vi "stimulate_and_record.vi"(3 "SSH password":string, 4 "Transfer and Run Date Folder After Experiment":bool, 5 "SSH user name":string, 6 "Tags":string, 7 "Frames":i32, 8 "Convert Power to Voltage":bool, 9 "voltages/power":dbl[](array[numeric]), 10 "parameters":string[](array[string]), 11 "parameters headers":string[](array[string])) -> ()   [LabVIEW 2014]
uses:
  <vilib>/userdefined/High Color/IMAQdx.ctl
  <vilib>/Utility/file.llb/Write To Spreadsheet File (string).vi
  <vilib>/Utility/file.llb/Read From Spreadsheet File (string).vi
  <vilib>/Utility/file.llb/Write To Spreadsheet File (DBL).vi
panel:
  out "Error":string
  out "Save Directory":path
  out "Buffer Number Out":u32
  out "Image":T1(plugin-control)
  in  "stop":bool
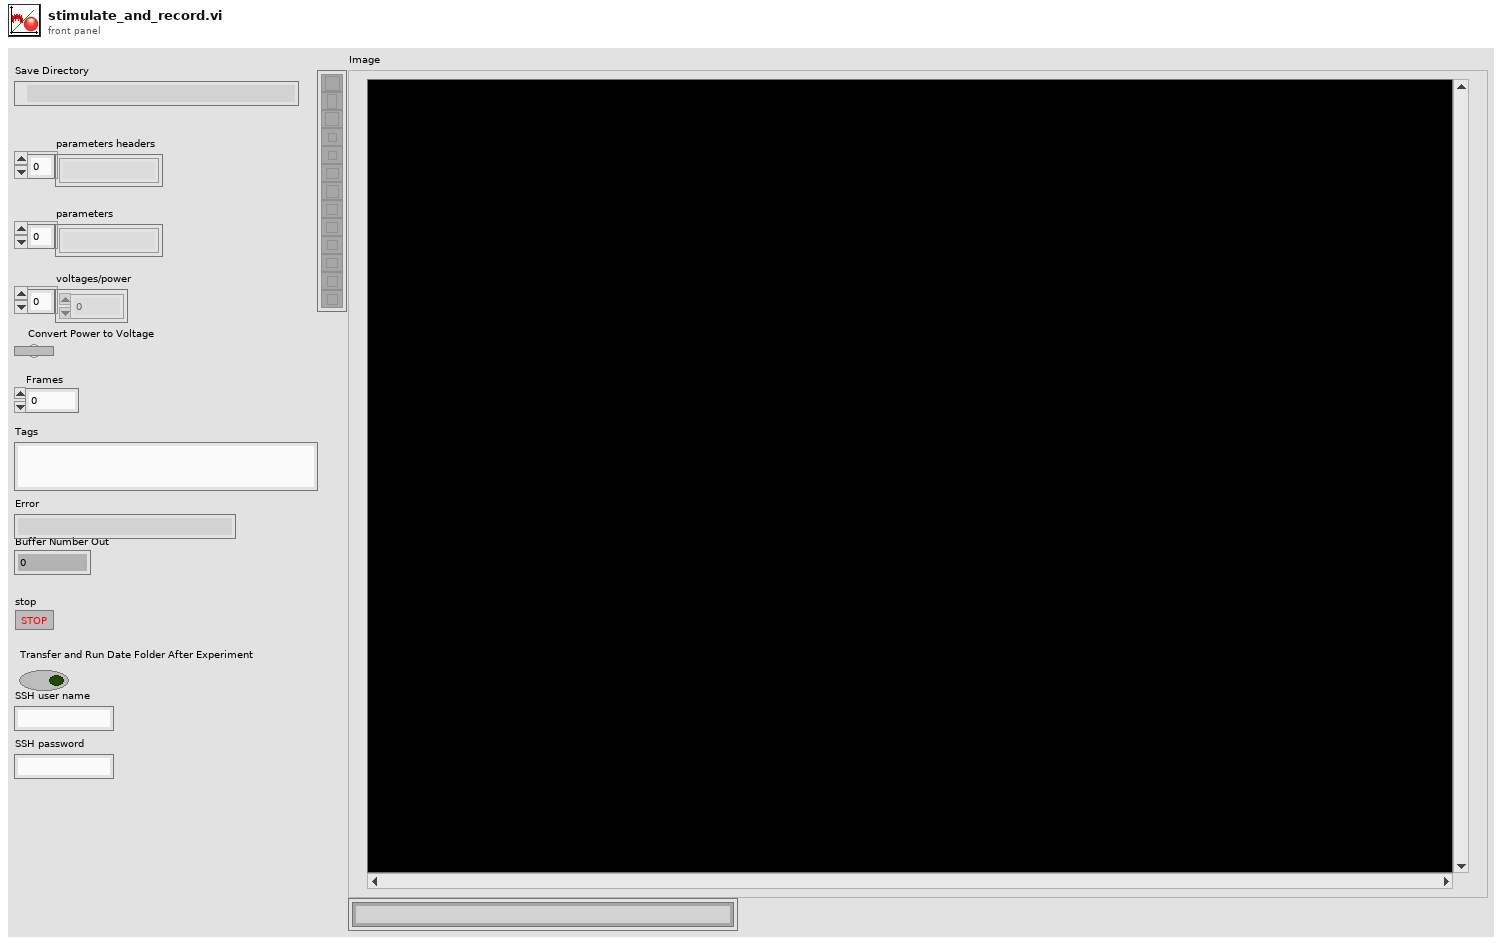
[diagram p1: front panel]
types:
  T1 = typedef "IMAQ Image.ctl" = refnum<image>
  T2 = typedef "IMAQdx.ctl" = refnum<k21>
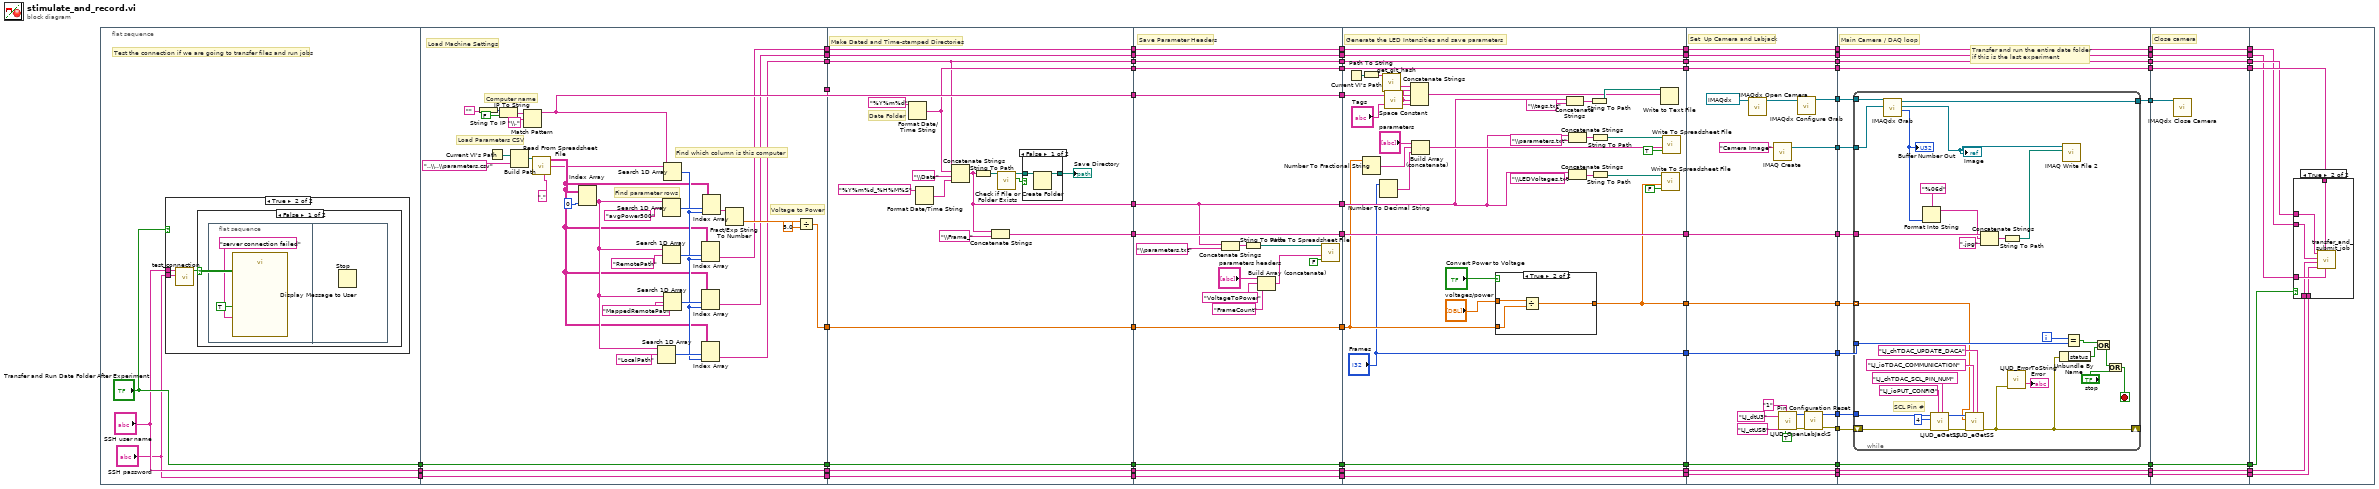
[diagram p0: block diagram]
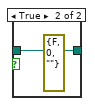
[diagram p4: hidden frame]
diagram:
  n1 = flat-sequence {
    tunnel: ["Transfer and Run Date Folder After Experiment"] -> w24
    tunnel: ["SSH user name"] -> w23
    tunnel: ["SSH password"] -> w22
    tunnel: [w105] -> w61
    tunnel: [w104] -> w60
    tunnel: [w91] -> w51
    tunnel: [w90] -> w50
    tunnel: [w89] -> w49
    tunnel: w24 -> [w83]
    tunnel: w23 -> [w82]
    tunnel: w22 -> [w81]
    tunnel: [w83] -> w15
    tunnel: [w82] -> w8
    tunnel: [w81] -> w7
    tunnel: [w133] -> w40
    tunnel: [w132] -> w38
    tunnel: [w131] -> w36
    tunnel: [w130] -> w34
    tunnel: [w129] -> w32
    tunnel: [w128] -> w30
    tunnel: [w127] -> w28
    tunnel: [w126] -> w26
    tunnel: w49 -> [w127]
    tunnel: w50 -> [w126]
    tunnel: w51 -> [w128]
    tunnel: w60 -> [w130]
    tunnel: w61 -> [w131]
    tunnel: [w116] -> w16
    tunnel: w15 -> [w116]
    tunnel: [w115] -> w9
    tunnel: w8 -> [w115]
    tunnel: w7 -> [w114]
    tunnel: [w114] -> w6
    tunnel: w40 -> [w155]
    tunnel: [w155] -> w39
    tunnel: w38 -> [w140]
    tunnel: [w140] -> w37
    tunnel: w36 -> [w154]
    tunnel: [w154] -> w35
    tunnel: w34 -> [w153]
    tunnel: [w153] -> w33
    tunnel: w32 -> [w152]
    tunnel: [w152] -> w31
    tunnel: w30 -> [w151]
    tunnel: [w151] -> w29
    tunnel: w28 -> [w150]
    tunnel: [w150] -> w27
    tunnel: w26 -> [w149]
    tunnel: [w149] -> w25
    tunnel: [w139] -> w17
    tunnel: w16 -> [w139]
    tunnel: [w138] -> w10
    tunnel: w9 -> [w138]
    tunnel: w6 -> [w137]
    tunnel: [w137] -> w5
    tunnel: w39 -> [w189]
    tunnel: [w189] -> w66
    tunnel: [w168] -> w64
    tunnel: ["Frames"] -> w63
    tunnel: w37 -> [w181]
    tunnel: w35 -> [w164]
    tunnel: w33 -> [w177]
    tunnel: w31 -> [w174]
    tunnel: [w174] -> w56
    tunnel: [w173] -> w52
    tunnel: w29 -> [w173]
    tunnel: [w172] -> w45
    tunnel: w27 -> [w172]
    tunnel: [w171] -> w41
    tunnel: w25 -> [w171]
    tunnel: [w162] -> w18
    tunnel: w17 -> [w162]
    tunnel: [w161] -> w11
    tunnel: w10 -> [w161]
    tunnel: w5 -> [w160]
    tunnel: [w160] -> w4
    tunnel: w66 -> [w213]
    tunnel: [w215] -> w72
    tunnel: [w214] -> w71
    tunnel: [w213] -> w70
    tunnel: [w205] -> w68
    tunnel: [w204] -> w67
    tunnel: [w209] -> w65
    tunnel: w64 -> [w209]
    tunnel: w63 -> [w208]
    tunnel: [w208] -> w62
    tunnel: [w202] -> w57
    tunnel: w56 -> [w202]
    tunnel: [w201] -> w53
    tunnel: w52 -> [w201]
    tunnel: [w200] -> w46
    tunnel: w45 -> [w200]
    tunnel: [w199] -> w42
    tunnel: w41 -> [w199]
    tunnel: [w198] -> w19
    tunnel: w18 -> [w198]
    tunnel: [w197] -> w12
    tunnel: w11 -> [w197]
    tunnel: w4 -> [w196]
    tunnel: [w196] -> w3
    tunnel: w72 -> [w233]
    tunnel: w71 -> [w232]
    tunnel: w70 -> [w231]
    tunnel: [w230] -> w69
    tunnel: w68 -> [w229]
    tunnel: w67 -> [w228]
    tunnel: w65 -> [w227]
    tunnel: w62 -> [w226]
    tunnel: [w225] -> w58
    tunnel: w57 -> [w225]
    tunnel: [w224] -> w54
    tunnel: w53 -> [w224]
    tunnel: [w223] -> w47
    tunnel: w46 -> [w223]
    tunnel: [w222] -> w43
    tunnel: w42 -> [w222]
    tunnel: [w221] -> w20
    tunnel: w19 -> [w221]
    tunnel: [w220] -> w13
    tunnel: w12 -> [w220]
    tunnel: w3 -> [w219]
    tunnel: [w219] -> w2
    tunnel: w69 -> [w271]
    tunnel: [w270] -> w59
    tunnel: w58 -> [w270]
    tunnel: [w269] -> w55
    tunnel: w54 -> [w269]
    tunnel: [w268] -> w48
    tunnel: w47 -> [w268]
    tunnel: [w267] -> w44
    tunnel: w43 -> [w267]
    tunnel: [w266] -> w21
    tunnel: w20 -> [w266]
    tunnel: [w265] -> w14
    tunnel: w13 -> [w265]
    tunnel: w2 -> [w264]
    tunnel: [w264] -> w1
    tunnel: w59 -> [w278]
    tunnel: w55 -> [w277]
    tunnel: w48 -> [w275]
    tunnel: w44 -> [w276]
    tunnel: w21 -> [w274]
    tunnel: w14 -> [w273]
    tunnel: w1 -> [w272]
    frame #0 {
      # "Test the connection if we are going to transfer files and run jobs"
      n2 = case shown="True" "Transfer and Run Date Folder After Experiment" {
        tunnel: "SSH password" -> [_ w78]
        tunnel: "SSH user name" -> [_ w76]
        frame False {
        }
        frame True {
          n3 = call "test_connection.vi"("Username"=w76, "Password"=w78) -> ("Connection Successful"=w77:bool)  [unwired: 7 in]
          n4 = case shown="False" w77 {
            frame False {
              n5 = flat-sequence {
                frame #0 {
                  n6 = call "Display Message to User"("Enable"=TRUE, "Message"="server connection failed") -> ()  [unwired: 8 in, 2 out]
                }
                frame #1 {
                  n7 = Stop() -> ()  [unwired: 1 in]
                }
              }
            }
            frame True {
            }
          }
        }
      }
    }
    frame #1 {
      # "Find parameter rows"
      # "Find which column is this computer"
      # "Voltage to Power"
      # "Load Parameters CSV"
      # "Computer name"
      # "Load Machine Settings"
      n8 = String To IP(1:"") -> (0:w113:u32)
      n9 = Current VI's Path() -> (path=w108:path)
      n10 = IP To String(1:FALSE, 2:w113) -> (0:w110:string)
      n11 = Build Path(base path=w108, name or relative path="..\\..\\parameters.csv") -> (appended path=w87:path)
      n12 = Match Pattern(string=w110, regular expression="\\.") -> (before substring=w104:string)  [unwired: 1 in, 3 out]
      n13 = call-poly <vilib>:"Read From Spreadsheet File.vi"("delimiter (\\t)"=",", "file path (dialog if empty)"=w87) -> ("first row"=w85:string[], "all rows"=w86:string[][])  [unwired: 5 in, 3 out]
      n14 = Index Array(array=w86, index (col)=0) -> (element=w88:string[])  [unwired: 1 in]
      n15 = Search 1D Array(1D array=w88, element="LocalPath") -> (index of element=w93:i32)  [unwired: 1 in]
      n16 = Search 1D Array(1D array=w88, element="RemotePath") -> (index of element=w98:i32)  [unwired: 1 in]
      n17 = Search 1D Array(1D array=w88, element="avgPower500") -> (index of element=w99:i32)  [unwired: 1 in]
      n18 = Search 1D Array(1D array=w85, element=w104) -> (index of element=w92:i32)  [unwired: 1 in]
      n19 = Search 1D Array(1D array=w88, element="MappedRemotePath") -> (index of element=w97:i32)  [unwired: 1 in]
      n20 = Index Array(array=w86, index (row)=w98, index (col)=w92) -> (element=w89:string)
      n21 = Index Array(array=w86, index (row)=w97, index (col)=w92) -> (element=w90:string)
      n22 = Index Array(array=w86, index (row)=w93, index (col)=w92) -> (element=w91:string)
      n23 = Index Array(array=w86, index (row)=w99, index (col)=w92) -> (element=w96:string)
      n24 = Fract/Exp String To Number(string=w96) -> (number=w95:dbl)  [unwired: 3 in, 1 out]
      n25 = Divide(x=w95, y=5.0) -> (x/y=w105:dbl)
    }
    frame #2 {
      # "Date Folder"
      # "Make Dated and Time-stamped Directories"
      n26 = Format Date/Time String(time format string (%c)="%Y%m%d") -> (date/time string=w129:string)  [unwired: 2 in]
      n27 = Format Date/Time String(time format string (%c)="%Y%m%d_%H%M%S") -> (date/time string=w120:string)  [unwired: 2 in]
      n28 = Concatenate Strings(w128, w129, "\\Data", w120) -> (w132:string)
      n29 = String To Path(string=w132) -> (path=w119:path)
      n30 = Concatenate Strings(w132, "\\Frame_") -> (w133:string)
      n31 = call <vilib>:"Check if File or Folder Exists.vi"("path"=w119) -> ("file or folder exists?"=w124:bool, "dup path"=w123:path)  [unwired: 8 in, 1 out]
      n32 = case shown="False" w124 {
        tunnel: [w134 w136] -> w118
        tunnel: w123 -> [w135 w136]
        frame False {
          n33 = Create Folder(path (use dialog)=w135) -> (created path=w134:path)  [unwired: 2 in, 2 out]
        }
        frame True {
          (unwired) errorcluster {"status"=FALSE, "code"=0, "source"=""} ("error out")
        }
      }
      "Save Directory" <- w118
    }
    frame #3 {
      # "Save Parameter Headers"
      n34 = Concatenate Strings(w140, "\\parameters.txt") -> (w148:string)
      n35 = String To Path(string=w148) -> (path=w147:path)
      n36 = Build Array (concatenate)("parameters headers", "VoltageToPower", "FrameCount") -> (w144:string[])
      n37 = call-poly <vilib>:"Write To Spreadsheet File.vi"("append to file? (new file:F)"=FALSE, "1D data"=w144, "file path (dialog if empty)"=w147) -> ()  [unwired: 5 in, 1 out]
    }
    frame #4 {
      # "Generate the LED Intensities and save parameters"
      n38 = Current VI's Path() -> (path=w158:path)
      n39 = Path To String(path=w158) -> (string=w159:string)
      n40 = Number To Fractional String(number=w164) -> (F-format string=w165:string)  [unwired: 3 in]
      n41 = Number To Decimal String(number="Frames") -> (decimal integer string=w166:string)  [unwired: 1 in]
      n42 = call "get_git_hash.vi"("VI folder"=w159) -> ("github hash"=w156:string)  [unwired: 10 in]
      n43 = call <vilib>:"Space Constant.vi"() -> ("String"=w157:string)
      n44 = Concatenate Strings(w156, w157, w177, w157, "Tags") -> (w175:string)
      n45 = Build Array (concatenate)("parameters", w165, w166) -> (w182:string[])
      n46 = case shown="True" "Convert Power to Voltage" {
        tunnel: "voltages/power" -> [w192 w195]
        tunnel: [w192 w193] -> w168
        tunnel: w164 -> [_ w194]
        frame False {
        }
        frame True {
          n47 = Divide(x=w195, y=w194) -> (x/y=w193:dbl[])
        }
      }
      n48 = Concatenate Strings(w181, "\\tags.txt") -> (w179:string)
      n49 = Concatenate Strings(w181, "\\LEDVoltages.txt") -> (w191:string)
      n50 = Concatenate Strings(w181, "\\parameters.txt") -> (w186:string)
      n51 = String To Path(string=w179) -> (path=w178:path)
      n52 = String To Path(string=w191) -> (path=w190:path)
      n53 = String To Path(string=w186) -> (path=w185:path)
      n54 = Write to Text File(file (use dialog)=w178, text=w175) -> ()  [unwired: 2 in, 3 out]
      n55 = call-poly <vilib>:"Write To Spreadsheet File.vi"("append to file? (new file:F)"=FALSE, "1D data"=w168, "file path (dialog if empty)"=w190) -> ()  [unwired: 5 in, 1 out]
      n56 = call-poly <vilib>:"Write To Spreadsheet File.vi"("append to file? (new file:F)"=TRUE, "1D data"=w182, "file path (dialog if empty)"=w185) -> ()  [unwired: 5 in, 1 out]
    }
    frame #5 {
      # "Set  Up Camera and Labjack"
      n57 = call <vilib>:"IMAQdx Open Camera.vi"("Session In"=T2 "cam0") -> ("Session Out"=w217:T2)  [unwired: 9 in, 1 out]
      n58 = call "IMAQ Create"("Image Name"="Camera Image") -> ("New Image"=w214:T1)  [unwired: 4 in, 1 out]
      n59 = call "LJUD_OpenLabJackS.vi"("FirstFound"=TRUE, "Address"="1" ("DeviceType"), "ConnectionType"="LJ_ctUSB", "DeviceType"="LJ_dtU3") -> ("error out"=w203:errorcluster, "Handle"=w206:i32)  [unwired: 5 in, 1 out]
      n60 = call <vilib>:"IMAQdx Configure Grab.vi"("Session In"=w217) -> ("Session Out"=w215:T2)  [unwired: 9 in, 1 out]
      n61 = call "Pin Configuration Reset.vi"("error in"=w203, "Handle In"=w206) -> ("error out"=w204:errorcluster, "Handle Out"=w205:i32)  [unwired: 8 in]
    }
    frame #6 {
      # "Transfer and run the entire date folder\nif this is the last experiment"
      # "Main Camera / DAQ loop"
      n62 = while {
        tunnel: w233 -> [w263]
        tunnel: [w262] -> w230
        tunnel: w232 -> [w261]
        tunnel: w231 -> [w259]
        tunnel: w229 -> [w236]
        shift-right: [w237] -> _
        shift-left: w228 -> [w235]
        tunnel: w227 -> [w234] mode=indexing
        tunnel: w226 -> [w245]
        i -> [w246]
        stop <- w252 stop-if-true
        # "SCL Pin #"
        n63 = call <vilib>:"IMAQdx Grab.vi"("Image In"=w261, "Session In"=w263) -> ("Buffer Number Out"=w255:u32, "Image Out"=w260:T1, "Session Out"=w262:T2)  [unwired: 6 in, 1 out]
        "Image" <- w260
        "Buffer Number Out" <- w255
        n64 = Format Into String(format string="%06d" ("string"), w255) -> (resulting string=w254:string)  [unwired: 2 in, 1 out]
        n65 = call "LJUD_eGetSS.vi"("Channel"="LJ_chTDAC_SCL_PIN_NUM", "IOType"="LJ_ioPUT_CONFIG", "error in"=w235, "Value Write"=4, "Handle In"=w236) -> ("error out"=w238:errorcluster, "Handle Out"=w241:i32)  [unwired: 4 in, 1 out]
        n66 = call "LJUD_eGetSS.vi"("Channel"="LJ_chTDAC_UPDATE_DACA", "IOType"="LJ_ioTDAC_COMMUNICATION", "error in"=w238, "Value Write"=w234, "Handle In"=w241) -> ("error out"=w237:errorcluster)  [unwired: 4 in, 2 out]
        n67 = Concatenate Strings(w259, w254, ".jpg" ("string")) -> (w257:string)
        n68 = String To Path(string=w257) -> (path=w256:path)
        n69 = call "LJUD_ErrorToString.vi"("error in"=w237) -> ("String"=→"Error":string)  [unwired: 10 in]
        n70 = Unbundle By Name(w237) -> ("status"=w249:bool)
        n71 = call-poly "IMAQ Write File 2"("File Path"=w256, "Image"=w260) -> ()  [unwired: 8 in, 2 out]
        n72 = Equal?(x=w246, y=w245) -> (x = y?=w248:bool)
        n73 = Or(x=w248, y=w249) -> (x .or. y?=w247:bool)
        n74 = Or(x=w247, y="stop") -> (x .or. y?=w252:bool)
      }
    }
    frame #7 {
      # "Close camera"
      n75 = call <vilib>:"IMAQdx Close Camera.vi"("Session In"=w271) -> ()  [unwired: 10 in, 1 out]
    }
    frame #8 {
      n76 = case shown="True" w274 {
        tunnel: w278 -> [_ w284]
        tunnel: w277 -> [_ w283]
        tunnel: w276 -> [_ w282]
        tunnel: w275 -> [_ w281]
        tunnel: w273 -> [_ w280]
        tunnel: w272 -> [_ w279]
        frame False {
        }
        frame True {
          n77 = call "transfer_and_submit_job.vi"("Mapped Remote Directory Path"=w282, "Date Folder"=w284, "Password"=w279, "Username"=w280, "Remote Data Directory"=w281, "Local Data Directory"=w283) -> ()  [unwired: 6 in]
        }
      }
    }
  }
